vi "Teleop Drive subVI.vi"(9 "Buttons":bool[](array[boolean]), 10 "Axes":dbl[](array[numeric])) -> ()   [LabVIEW 2017]
doc: "This VI is called for each TeleOp packet received from the DS where the robot is not disabled. It is often used to read from the joysticks and update I/O or to update setpoints for timed control loops. It should complete and return within 20 milliseconds or it may miss DS packets."
uses:
  drive enum.ctl
  <vilib>/Rock Robotics/WPI/ThirdParty/Phoenix-LabVIEW/Motor Controller/Controls/CTRE_Phoenix_MotorControl_FeedbackDevice.ctl
  <vilib>/Rock Robotics/WPI/ThirdParty/Phoenix-LabVIEW/Motor Controller/Controls/CTRE_Phoenix_MotorControl_ControlMode.ctl
  <vilib>/Rock Robotics/WPI/Utilities/WPI_GetSetVariantRefNum.vi
  <vilib>/Rock Robotics/WPI/ThirdParty/Phoenix-LabVIEW/Motor Controller/Get/CTRE_Phoenix_MotorController_GetOutputCurrent_Enhanced.vi
  <vilib>/Rock Robotics/WPI/ThirdParty/Phoenix-LabVIEW/Motor Controller/Get/CTRE_Phoenix_MotorController_GetVoltage.vi
  <vilib>/Rock Robotics/WPI/ThirdParty/Phoenix-LabVIEW/Motor Controller/Get/CTRE_Phoenix_MotorController_GetClosedLoopData.vi
  <vilib>/Rock Robotics/WPI/ThirdParty/Phoenix-LabVIEW/Motor Controller/Get/CTRE_Phoenix_MotorController_GetSelectedSensorData.vi
  <vilib>/Rock Robotics/Network Tables/NT Write Variant.vi
  <vilib>/Rock Robotics/WPI/Solenoid/WPI_SolenoidSetEnum.vi
  <vilib>/Rock Robotics/WPI/Solenoid/WPI_SolenoidValue.ctl
panel:
  in  "X and Y values In":bool=TRUE
  in  "Tab Control":T1(tab)
  in  "Cruise Velocity 3":i32=2000
  in  "Max Acceleration 3":i32=2000
  in  "Cruise Velocity 4":i32=2000
  in  "Max Acceleration 4":i32=2000
  in  "P 3":dbl format="%#_13g"
  in  "I 3":dbl format="%#_13g"
  in  "D 3":dbl format="%#_13g"
  in  "F 3":dbl=0.0095 format="%#_13g"
  in  "P 4":dbl format="%#_13g"
  in  "I 4":dbl format="%#_13g"
  in  "D 4":dbl format="%#_13g"
  in  "F 4":dbl=0.0095 format="%#_13g"
  out "Velocity (Raw Sensor Units per 100 ms) 6":i32
  out "Position (inches) 6":i32
  out "Percent Output 4":dbl
  out "Velocity (Raw Sensor Units per 100 ms) 5":i32
  out "Position (Raw Sensor Units) 5":i32
  out "Percent Output 3":dbl
  out "Output Current 3":dbl
  out "Closed-loop Error 4":i32
  out "Output Current 4":dbl
  out "Closed-loop Error 3":i32
  out "Position (inches) 5":i32
  out "Position (Raw Sensor Units) 6":i32
  in  "P":dbl format="%#_13g"
  in  "I":dbl format="%#_13g"
  in  "D":dbl format="%#_13g"
  in  "F":dbl=0.0095 format="%#_13g"
  in  "Cruise Velocity":i32=2000
  in  "Max Acceleration":i32=2000
  in  "Cruise Velocity 2":i32=2000
  in  "Max Acceleration 2":i32=2000
  in  "P 2":dbl format="%#_13g"
  in  "I 2":dbl format="%#_13g"
  in  "D 2":dbl format="%#_13g"
  in  "F 2":dbl=0.0095 format="%#_13g"
  out "Closed-loop Error 2":i32
  out "Percent Output 2":dbl
  out "Output Current 2":dbl
  out "Velocity (Raw Sensor Units per 100 ms) 4":i32
  out "Position (Raw Sensor Units) 4":i32
  out "Percent Output":dbl
  out "Output Current":dbl
  out "Velocity (Raw Sensor Units per 100 ms) 3":i32
  out "Position (Raw Sensor Units) 3":i32
  out "Closed-loop Error":i32
  out "Velocity (Raw Sensor Units per 100 ms) 7":i32
  out "Position (Raw Sensor Units) 7":i32
  out "Closed-loop Error 5":i32
  out "Percent Output 5":dbl
  out "Output Current 5":dbl
  out "Closed-loop Error 6":i32
  in  "Cruise Velocity 5":i32=2000
  in  "Max Acceleration 5":i32=2000
  in  "Cruise Velocity 6":i32=2000
  in  "Max Acceleration 6":i32=2000
  in  "P 5":dbl format="%#_13g"
  in  "D 5":dbl format="%#_13g"
  in  "F 5":dbl=0.0095 format="%#_13g"
  in  "I 5":dbl format="%#_13g"
  in  "P 6":dbl format="%#_13g"
  in  "I 6":dbl format="%#_13g"
  in  "D 6":dbl format="%#_13g"
  in  "F 6":dbl=0.0095 format="%#_13g"
  out "Velocity (Raw Sensor Units per 100 ms) 8":i32
  out "Position (Raw Sensor Units) 8":i32
  out "Percent Output 6":dbl
  out "Output Current 6":dbl
  out "Position (Raw Sensor Units)":i32
  out "Velocity (Raw Sensor Units per 100 ms)":i32
  out "Position (Raw Sensor Units) 2":i32
  out "Velocity (Raw Sensor Units per 100 ms) 2":i32
  in  "X axis value":dbl
  in  "Y axis value":dbl
  out "encoder position":i32(graph)
  out "X and Y":T2(graph)
  out "joystick X":dbl
  out "joystick Y":dbl
  out "closed loop error":T3(graph)
  out "voltage vs current left":T2(graph)
  out "voltage vs current right":T2(graph)
  out "Speed Closed Loop Plots":T4(graph)
  # "front panel"
  # "joystick"
  # "what we want"
  # "actual"
  # "0.005740418607"
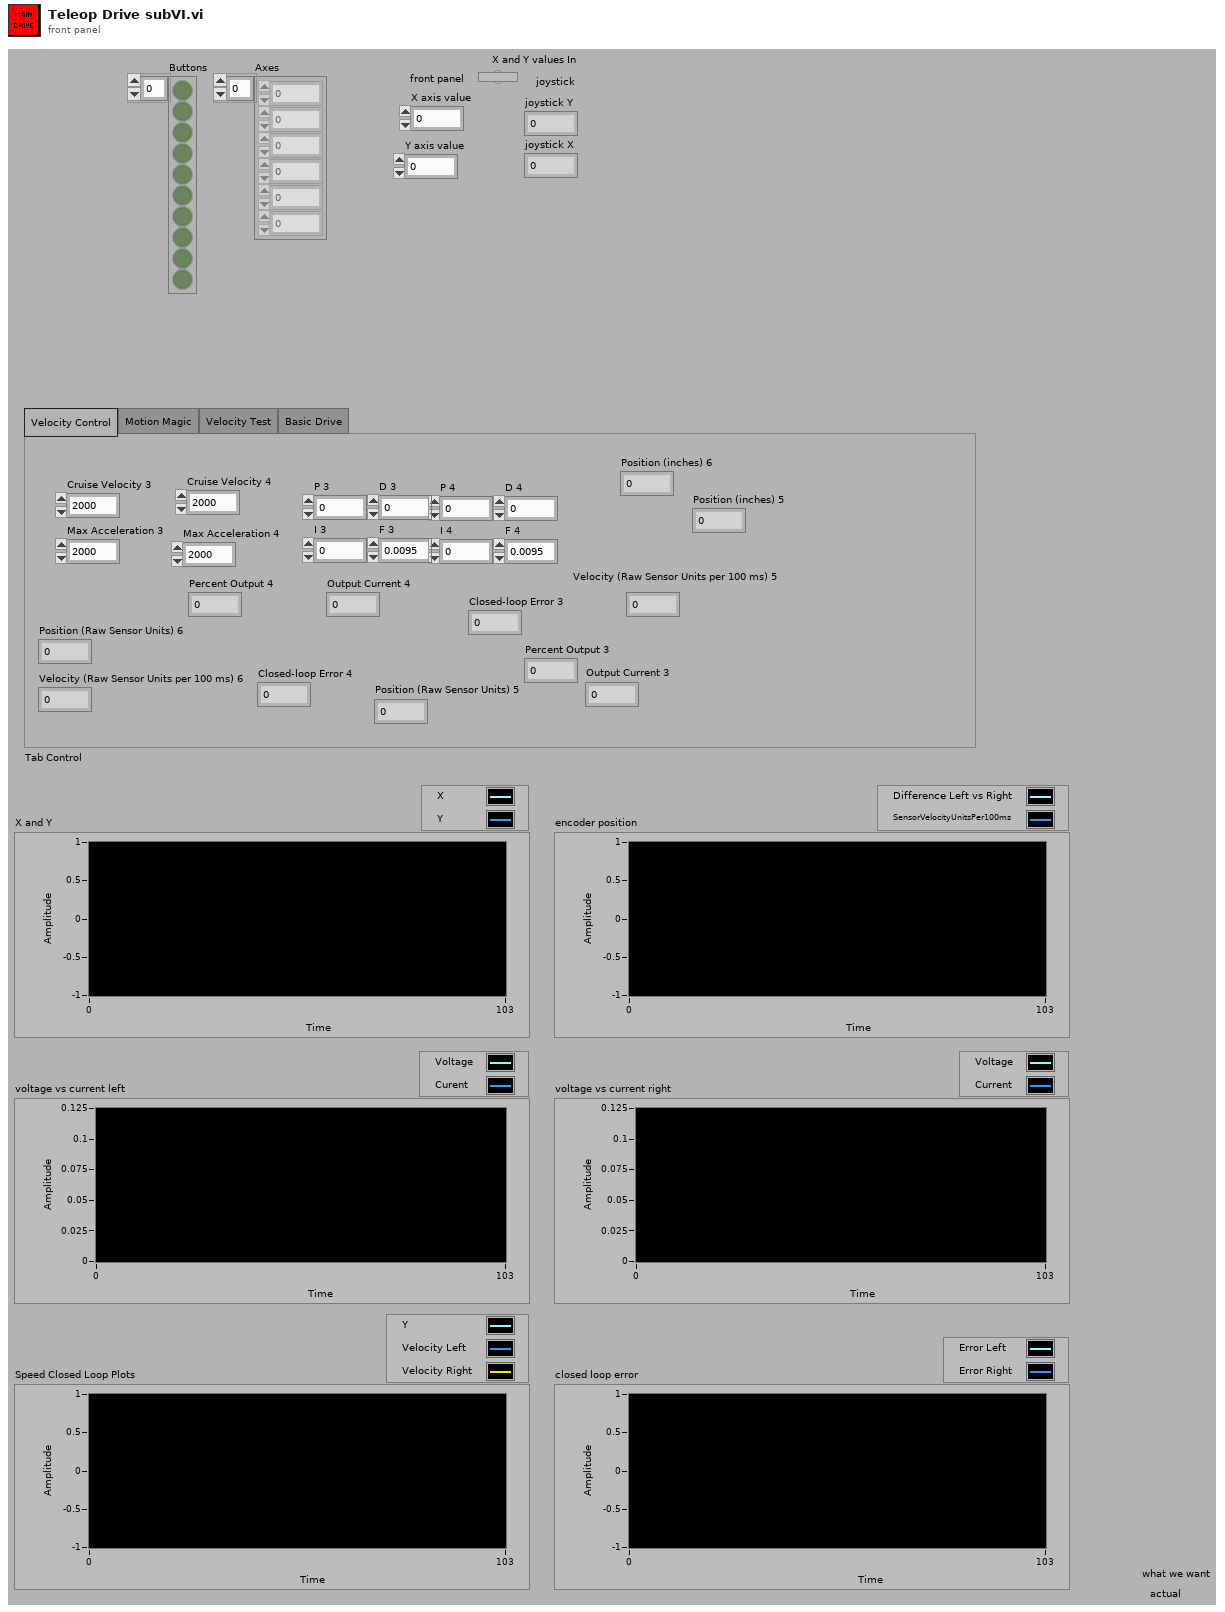
[diagram p1: front panel]
types:
  T1 = enum32{"Velocity Control", "Motion Magic", "Velocity Test", "Basic Drive"}
  T2 = cluster{"Percent Output":dbl, "Output Current":dbl}
  T3 = cluster{"Closed-loop Error":i32, "Closed-loop Error":i32}
  T4 = cluster{dbl, "Velocity (Raw Sensor Units per 100 ms)":i32, "Velocity (Raw Sensor Units per 100 ms)":i32}
  T5 = typedef "drive enum.ctl" = enum16{"Velocity Control", "Motion Magic", "Velocity Test", "Basic Drive"}
  T6 = typedef "WPI_SolenoidValue.ctl" = enum16{"Off", "On", "Forward", "Reverse"}
  T7 = typedef "WPI_SolenoidDevRef.ctl" = cluster{"DevStatus":errorcluster, "Pneumatics Control Module":u8, "Forward Solenoid Channel":T8, "Reverse Solenoid Channel":T8}
  T8 = typedef "WPI_SolenoidChannel.ctl" = enum8{"Solenoid 0", "Solenoid 1", "Solenoid 2", "Solenoid 3", "Solenoid 4", "Solenoid 5", "Solenoid 6", "Solenoid 7", "Invalid"}
  T9 = typedef "WPI_RobotDriveDevRef.ctl" = cluster{"DevStatus":errorcluster, "Motors[]":T10[], "Square Inputs":bool, "Max Output":dbl}
  T10 = typedef "WPI_MotorControlDeviceRef.ctl" = cluster{"DeviceStatus":errorcluster, "Type":T11, "PWM":cluster{"PWM Channel":T12, "DeadBand":T13}, "CAN":cluster{"Device Number":u8, "SetOutput VI Ref":variant, "GetOutput VI Ref":variant, "Enable VI Ref":variant, "Disable VI Ref":variant, "Data":variant}, "Invert":bool, "DIO PWM":cluster{"PWM \"Enable\" Channel":T12, "DIOChannel":T14, "PWM Rate":dbl}}
  T11 = typedef "WPI_MotorControlType.ctl" = enum16{"PWM", "CAN", "DIO PWM"}
  T12 = typedef "FPGA_DIOPWMChannel.ctl" = enum8{"PWM 0", "PWM 1", "PWM 2", "PWM 3", "PWM 4", "PWM 5", "PWM 6", "PWM 7", "PWM 8", "PWM 9", "PWM MXP 0", "PWM MXP 1", "PWM MXP 2", "PWM MXP 3", "PWM MXP 4", "PWM MXP 5", "PWM MXP 6", "PWM MXP 7", "PWM MXP 8", "PWM MXP 9", "Invalid"}
  T13 = typedef "WPI_PWMDeadband.ctl" = cluster{"Name":string, "maxPositivePwm":i32, "minPositivePwm":i32, "centerPwm":i32, "maxNegativePwm":i32, "minNegativePwm":i32, "angularRange":u16}
  T14 = typedef "FPGA_DIOChannel.ctl" = enum8{"DIO 0", "DIO 1", "DIO 2", "DIO 3", "DIO 4", "DIO 5", "DIO 6", "DIO 7", "DIO 8", "DIO 9", "DIO MXP 0", "DIO MXP 1", "DIO MXP 2", "DIO MXP 3", "DIO MXP 4", "DIO MXP 5", "DIO MXP 6", "DIO MXP 7", "DIO MXP 8", "DIO MXP 9", "DIO MXP 10", "DIO MXP 11", "DIO MXP 12", "DIO MXP 13", "DIO MXP 14", "DIO MXP 15", "SPI Port CS1", "SPI Port CS2", "SPI Port CS3", "SPI Port MISO", "SPI Port MOSI", "Invalid"}
  T15 = typedef "CTRE_Phoenix_MotorControl_ControlMode.ctl" = u16
  T16 = typedef "CTRE_Phoenix_MotorControl_FeedbackDevice.ctl" = i8
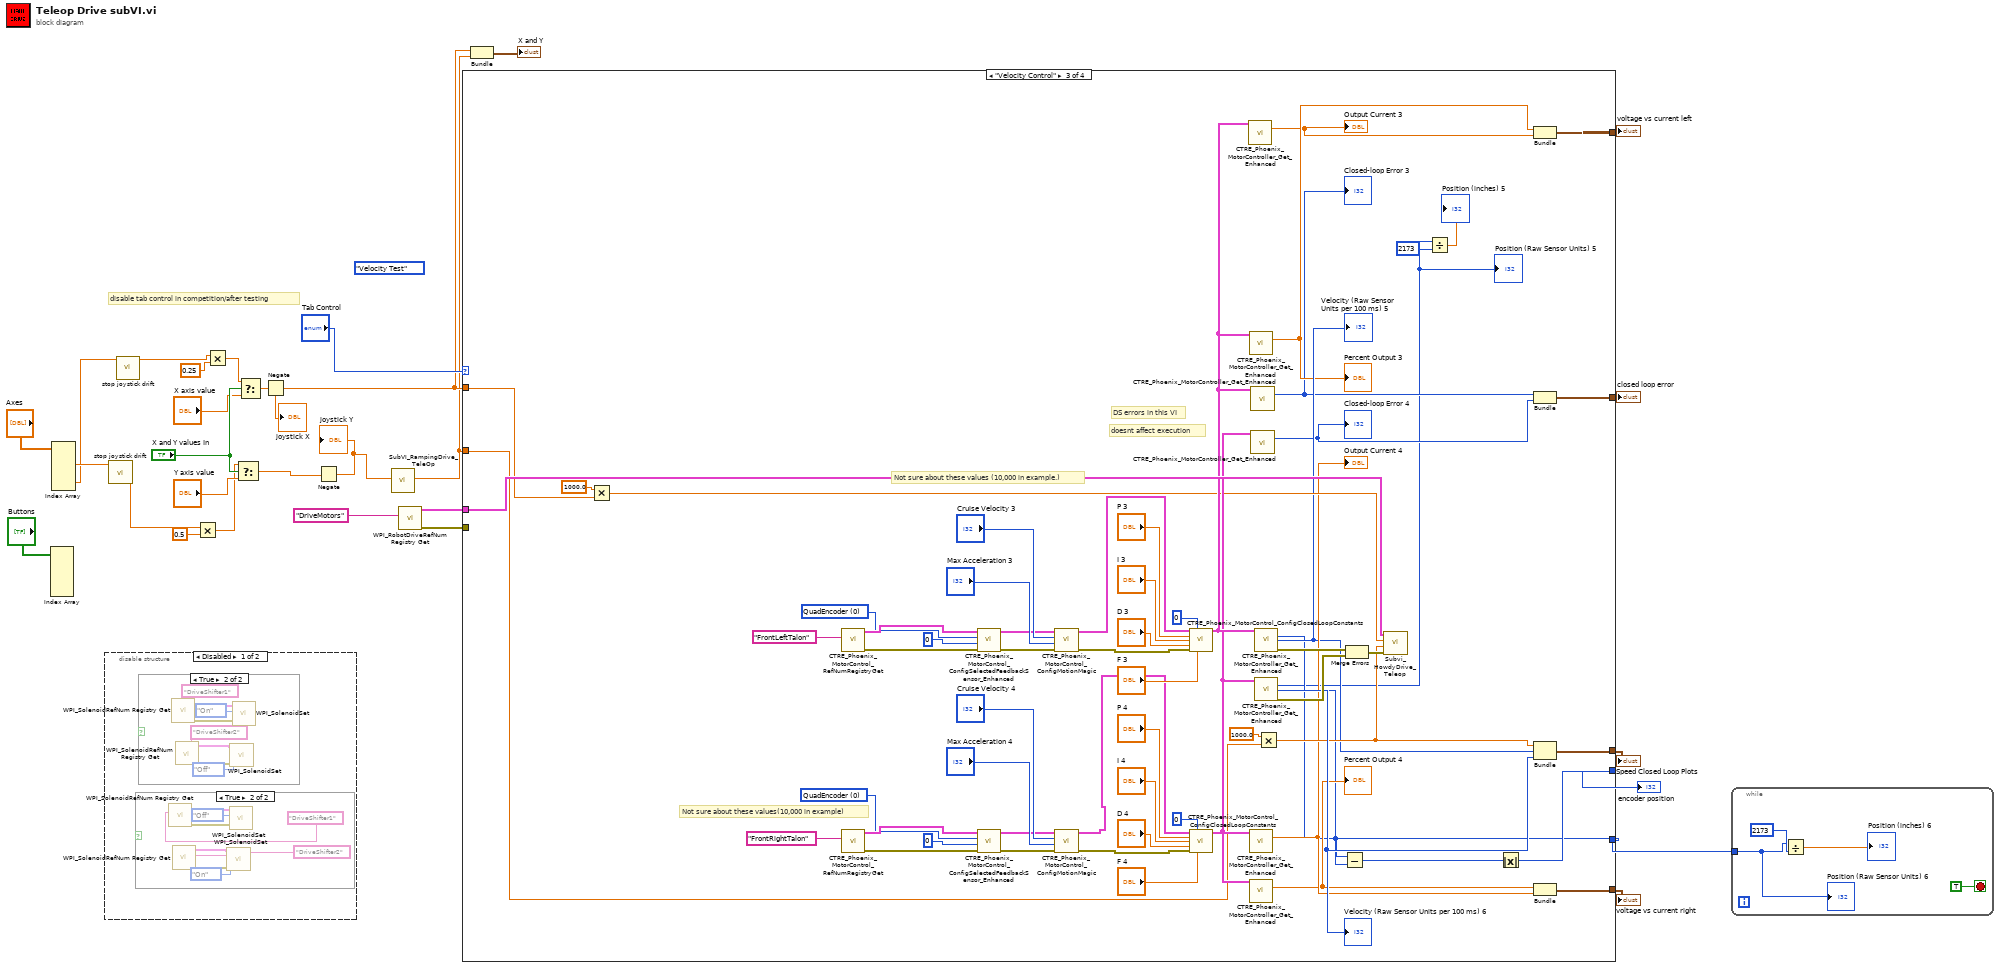
[diagram p0: block diagram]
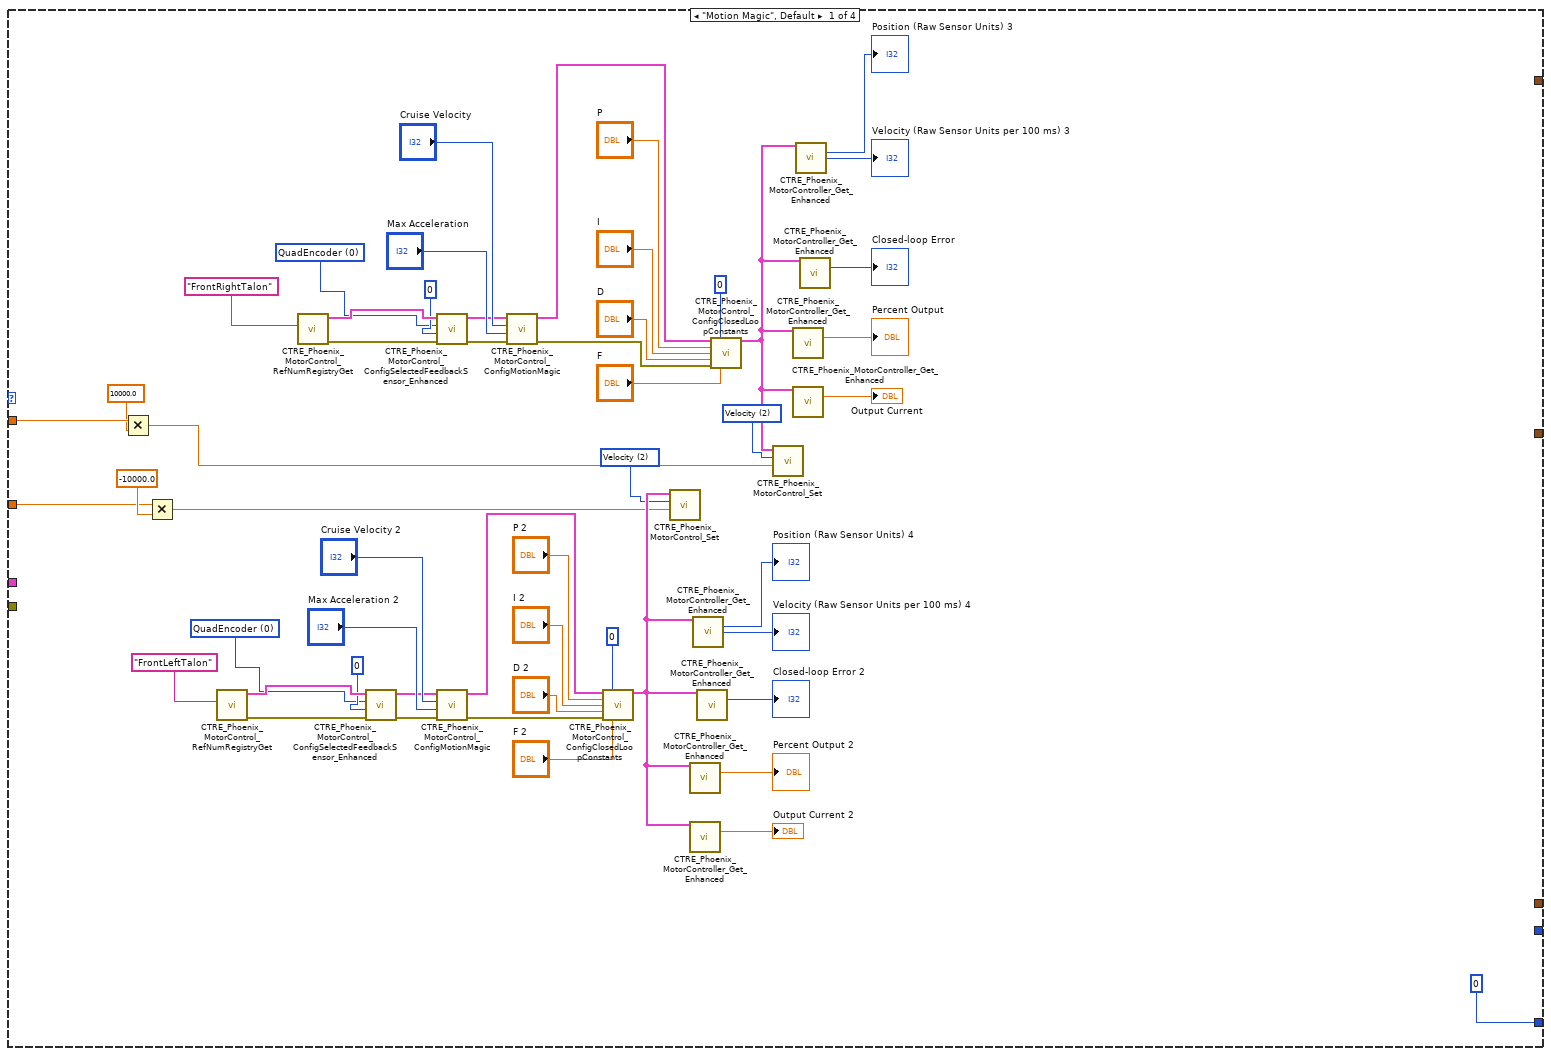
[diagram p5: hidden frame]
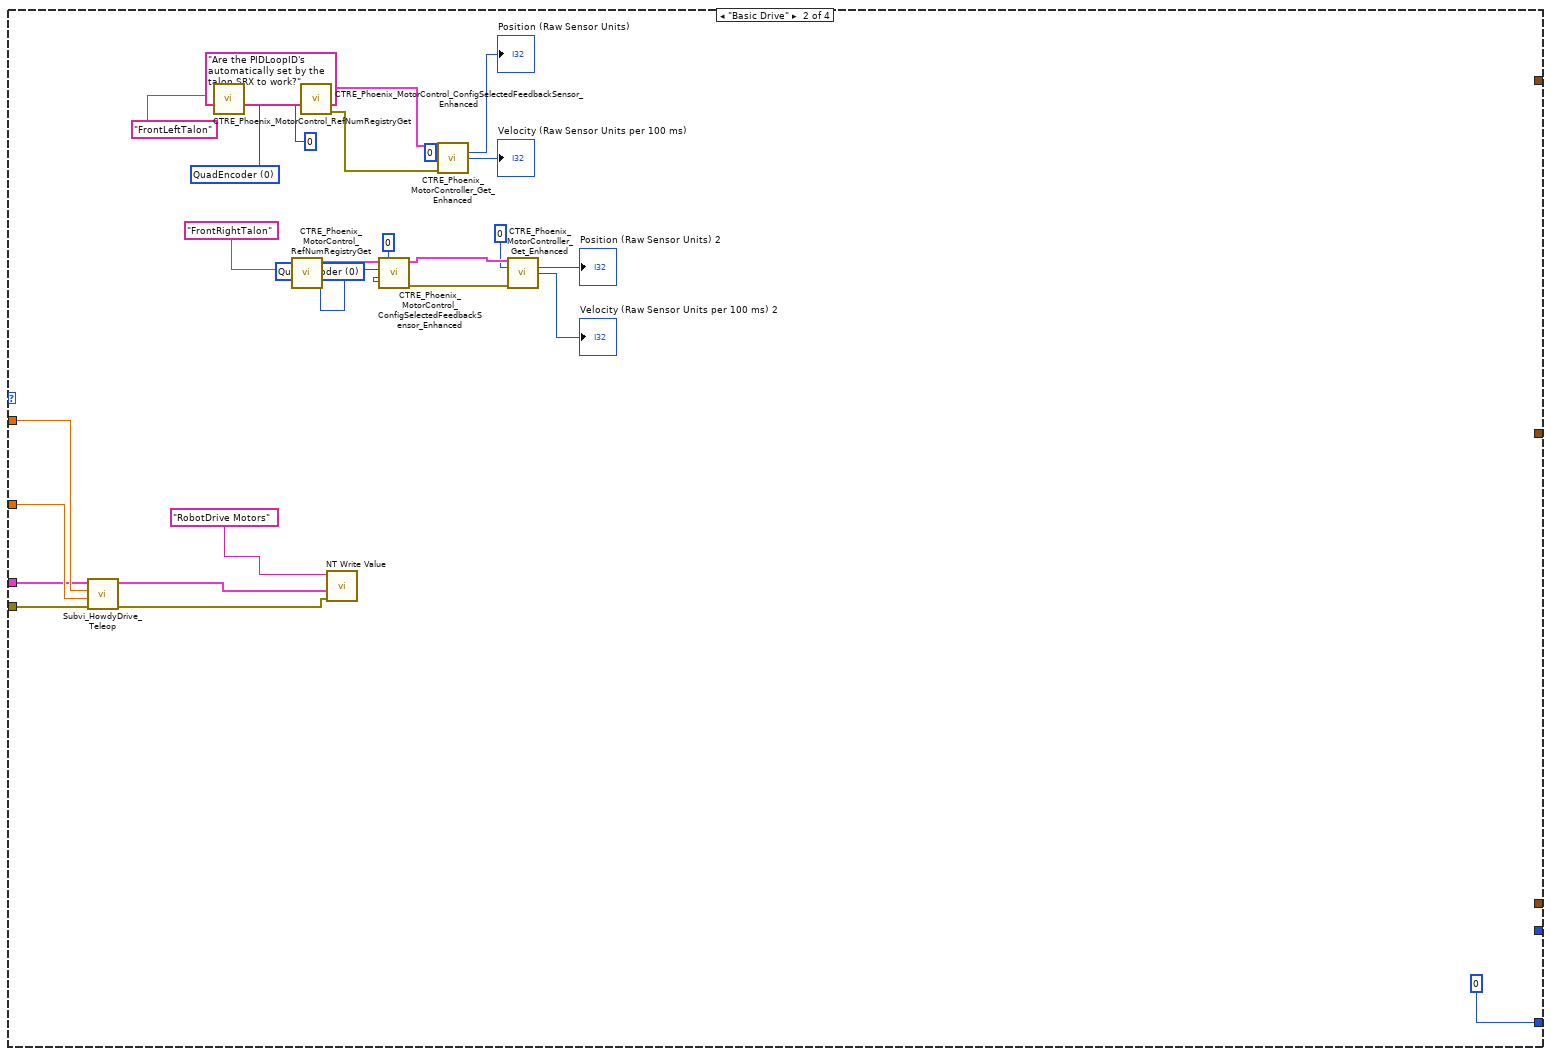
[diagram p6: hidden frame]
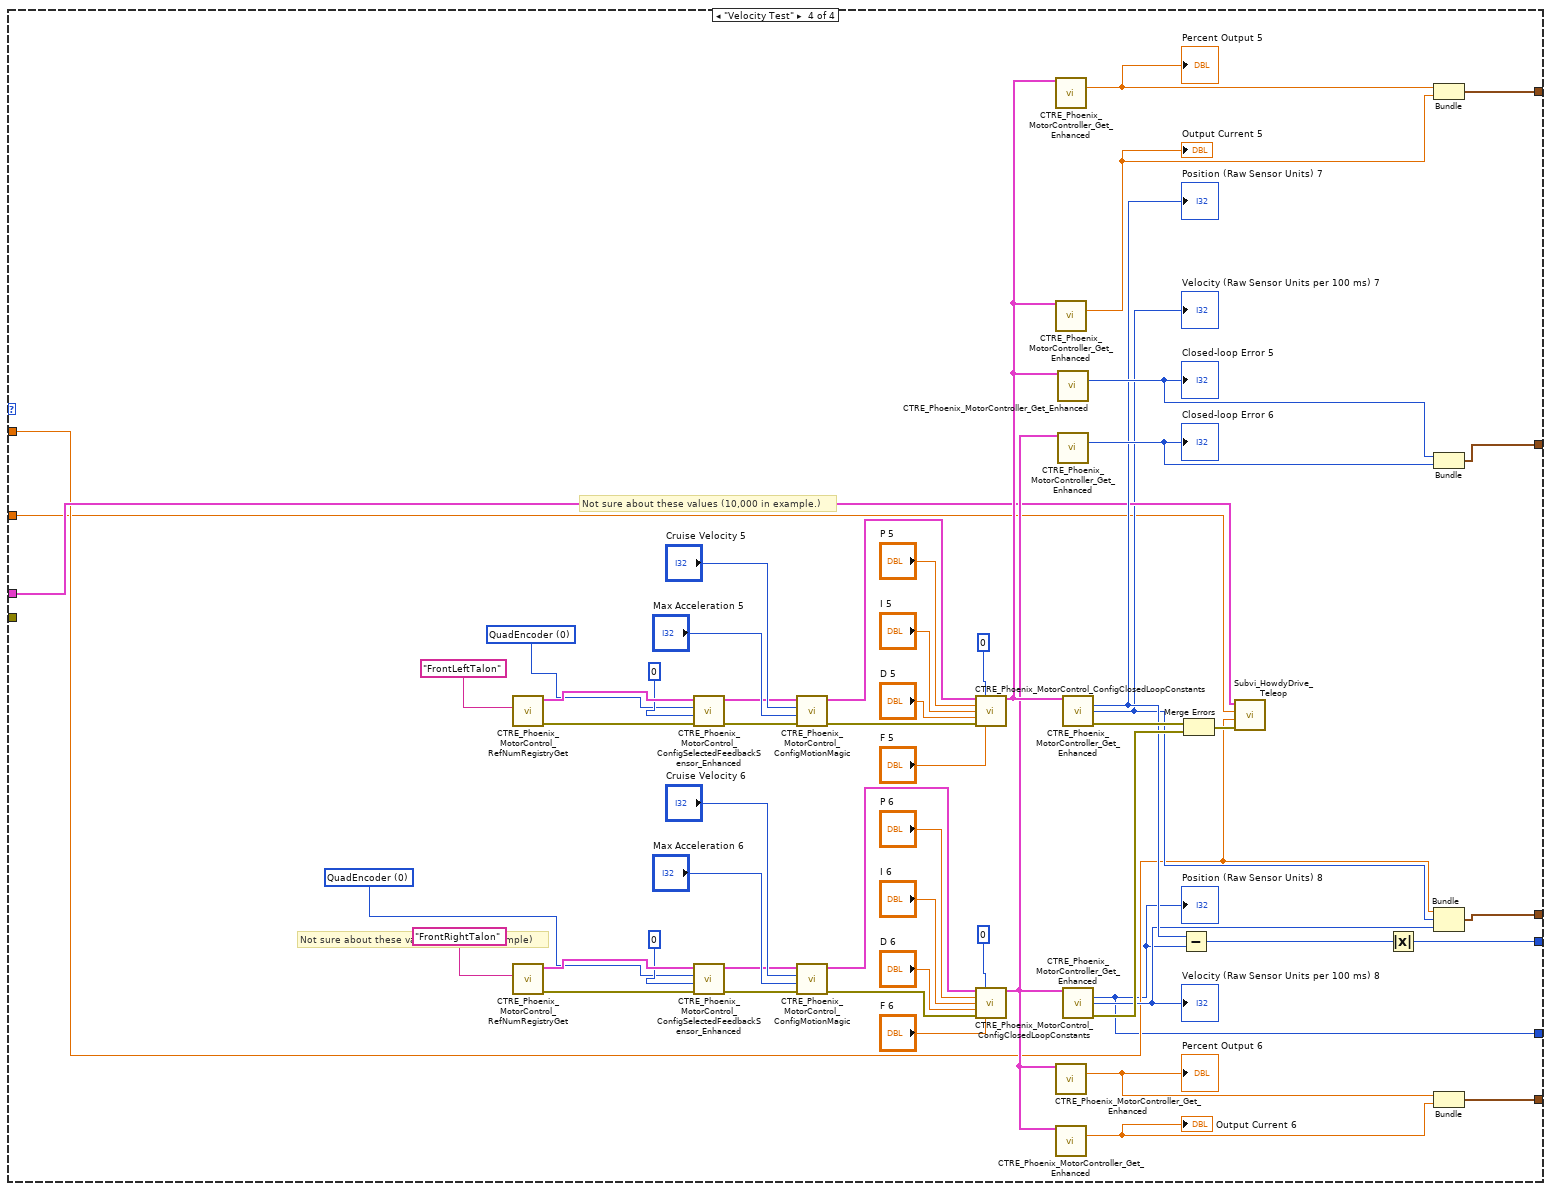
[diagram p7: hidden frame]
diagram:
  (unwired) drive_enum."Velocity Test"
  # "disable tab control in competition/after testing"
  n1 = Index Array(array="Buttons") -> ()  [unwired: 6 in, 6 out]
  n2 = Index Array(array="Axes") -> (element #2=w19:dbl, element #5=w12:dbl)  [unwired: 6 in, 4 out]
  n3 = disable-structure shown="Disabled" {
    frame Disabled {
      n4 = case shown="True" {
        selector: _ -> [_ _]
        frame False {
        }
        frame True {
          n5 = call <vilib>:"WPI_SolenoidRefNum Registry Get.vi"("refnum name"="DriveShifter1") -> ("error out"=w44:errorcluster, "SolenoidDevRef"=w45:T7)  [unwired: 9 in]
          n6 = call <vilib>:"WPI_SolenoidRefNum Registry Get.vi"("refnum name"="DriveShifter2") -> ("error out"=w42:errorcluster, "SolenoidDevRef"=w43:T7)  [unwired: 9 in]
          n7 = call-poly <vilib>:"WPI_SolenoidSet.vi"("error in (no error)"=w42, "Value"=WPI_SolenoidValue."On", "SolenoidDevRef"=w43) -> ()  [unwired: 7 in, 2 out]
          n8 = call-poly <vilib>:"WPI_SolenoidSet.vi"("error in (no error)"=w44, "Value"=WPI_SolenoidValue."Off", "SolenoidDevRef"=w45) -> ()  [unwired: 7 in, 2 out]
        }
      }
      n9 = case shown="True" {
        selector: _ -> [_ _]
        frame False {
        }
        frame True {
          n10 = call <vilib>:"WPI_SolenoidRefNum Registry Get.vi"("refnum name"="DriveShifter1") -> ("error out"=w36:errorcluster, "SolenoidDevRef"=w37:T7)  [unwired: 9 in]
          n11 = call <vilib>:"WPI_SolenoidRefNum Registry Get.vi"("refnum name"="DriveShifter2") -> ("error out"=w34:errorcluster, "SolenoidDevRef"=w35:T7)  [unwired: 9 in]
          n12 = call-poly <vilib>:"WPI_SolenoidSet.vi"("error in (no error)"=w34, "Value"=WPI_SolenoidValue."Off", "SolenoidDevRef"=w35) -> ()  [unwired: 7 in, 2 out]
          n13 = call-poly <vilib>:"WPI_SolenoidSet.vi"("error in (no error)"=w36, "Value"=WPI_SolenoidValue."On", "SolenoidDevRef"=w37) -> ()  [unwired: 7 in, 2 out]
        }
      }
    }
    frame Enabled {
    }
  }
  n14 = call "stop joystick drift.vi"("upper limit in"=w19) -> ("upper limit out"=w8:dbl)  [unwired: 10 in]
  n15 = call "stop joystick drift.vi"("upper limit in"=w12) -> ("upper limit out"=w10:dbl)  [unwired: 10 in]
  n16 = Multiply(x=w8, y=0.5) -> (x*y=w6:dbl)
  n17 = Multiply(x=w10, y=0.25) -> (x*y=w5:dbl)
  n18 = Select(t=w6, s="X and Y values In", f="Y axis value") -> (s? t:f=w16:dbl)
  n19 = Select(t=w5, s="X and Y values In", f="X axis value") -> (s? t:f=w17:dbl)
  n20 = Negate(x=w17) -> (-x=w13:dbl)
  "joystick X" <- w13
  n21 = Negate(x=w16) -> (-x=w1:dbl)
  "joystick Y" <- w1
  n22 = call "SubVI_RampingDrive_TeleOp.vi"("joystick Y Input"=w1) -> ("joystick Y Output"=w2:dbl)  [unwired: 9 in, 1 out]
  n23 = call <vilib>:"WPI_RobotDriveRefNum Registry Get.vi"("refnum name"="DriveMotors") -> ("error out"=w11:errorcluster, "RobotDriveDevRef"=w28:T9)  [unwired: 1 in, 8 out]
  n24 = case shown="\"Velocity Control\"" "Tab Control" {
    tunnel: w2 -> [w49 w123 w149 w188]
    tunnel: w13 -> [w52 w122 w150 w189]
    tunnel: w28 -> [_ w121 w186 w197]
    tunnel: [_ _ w137 w196] -> w26
    tunnel: [_ _ w135 w194] -> w25
    tunnel: [_ _ w134 w192] -> w24
    tunnel: [_ _ w133 w193] -> w23
    tunnel: [_ _ w136 w195] -> w22
    tunnel: w11 -> [_ w101 _ _]
    tunnel: [0 ("Position (Raw Sensor Units)") 0 ("Position (Raw Sensor Units)") w128 w187] -> w4
    frame "Motion Magic", Default {
      w57 = T15 2 items=["PercentOutput"=0, "Position"=1, "Velocity"=2, "Current"=3, "Follower"=5, "MotionProfile"=6, "MotionMagic"=7, "MotionMagicArc"=8, "MotionProfileArc"=10, "Disabled"=15] ("Control Mode")
      w54 = T16 0 items=["None"=-1, "QuadEncoder"=0, "Analog"=2, "Tachometer"=4, "Pulse Width Encoded Position"=8, "Sensor Sum (S0 + S1)"=9, "Sensor Difference (D0 - D1)"=10, "Remote Source 0"=11, "Remote Source 1"=12, "Software Emulated"=15] ("Feedback Device")
      w80 = T15 2 items=["PercentOutput"=0, "Position"=1, "Velocity"=2, "Current"=3, "Follower"=5, "MotionProfile"=6, "MotionMagic"=7, "MotionMagicArc"=8, "MotionProfileArc"=10, "Disabled"=15] ("Control Mode")
      w77 = T16 0 items=["None"=-1, "QuadEncoder"=0, "Analog"=2, "Tachometer"=4, "Pulse Width Encoded Position"=8, "Sensor Sum (S0 + S1)"=9, "Sensor Difference (D0 - D1)"=10, "Remote Source 0"=11, "Remote Source 1"=12, "Software Emulated"=15] ("Feedback Device")
      n25 = Multiply(x=w52, y=10000.0) -> (x*y=w47:dbl)
      n26 = Multiply(x=w49, y=-10000.0) -> (x*y=w48:dbl)
      n27 = call <vilib>:"CTRE_Phoenix_MotorControl_RefNumRegistryGet.vi"("refnum name"="FrontLeftTalon") -> ("error out"=w82:errorcluster, "PhoenixMotorControlDevRef"=w81:T10)  [unwired: 9 in]
      n28 = call <vilib>:"CTRE_Phoenix_MotorControl_RefNumRegistryGet.vi"("refnum name"="FrontRightTalon") -> ("error out"=w59:errorcluster, "PhoenixMotorControlDevRef"=w58:T10)  [unwired: 9 in]
      n29 = call <vilib>:"CTRE_Phoenix_MotorControl_ConfigSelectedFeedbackSensor_Enhanced.vi"("error in (no error)"=w82, "pidLoopIdx"=0, "Feedback Device"=w77, "PhoenixMotorControlDevRef"=w81) -> ("error out"=w84:errorcluster, "PhoenixMotorControlDevRef"=w83:T10)  [unwired: 6 in]
      n30 = call <vilib>:"CTRE_Phoenix_MotorControl_ConfigSelectedFeedbackSensor_Enhanced.vi"("error in (no error)"=w59, "pidLoopIdx"=0, "Feedback Device"=w54, "PhoenixMotorControlDevRef"=w58) -> ("error out"=w61:errorcluster, "PhoenixMotorControlDevRef"=w60:T10)  [unwired: 6 in]
      n31 = call <vilib>:"CTRE_Phoenix_MotorControl_ConfigMotionMagic.vi"("error in (no error)"=w84, "Acceleration"="Max Acceleration 2", "Cruise Velocity"="Cruise Velocity 2", "PhoenixMotorControlDevRef"=w83) -> ("error out"=w95:errorcluster, "PhoenixMotorControlDevRef"=w94:T10)  [unwired: 6 in]
      n32 = call <vilib>:"CTRE_Phoenix_MotorControl_ConfigMotionMagic.vi"("error in (no error)"=w61, "Acceleration"="Max Acceleration", "Cruise Velocity"="Cruise Velocity", "PhoenixMotorControlDevRef"=w60) -> ("error out"=w63:errorcluster, "PhoenixMotorControlDevRef"=w62:T10)  [unwired: 6 in]
      n33 = call <vilib>:"CTRE_Phoenix_MotorControl_ConfigClosedLoopConstants.vi"("PhoenixMotorControlDevRef"=w94, "slotIdx"=0, "P"="P 2", "I"="I 2", "D"="D 2", "error in (no error)"=w95, "F"="F 2") -> ("PhoenixMotorControlDevRef"=w98:T10)  [unwired: 7 in, 1 out]
      n34 = call <vilib>:"CTRE_Phoenix_MotorControl_Set.vi"("Output"=w48, "Control Mode"=w80, "PhoenixMotorControlDevRef"=w98) -> ()  [unwired: 7 in, 2 out]
      n35 = call-poly <vilib>:"CTRE_Phoenix_MotorController_Get_Enhanced.vi"("PhoenixMotorControlDevRef"=w98) -> ("Percent Output"=→"Percent Output 2":dbl)  [unwired: 10 in, 4 out]
      n36 = call-poly <vilib>:"CTRE_Phoenix_MotorController_Get_Enhanced.vi"("PhoenixMotorControlDevRef"=w98) -> ("Output Current"=→"Output Current 2":dbl)  [unwired: 12 in, 2 out]
      n37 = call-poly <vilib>:"CTRE_Phoenix_MotorController_Get_Enhanced.vi"("PhoenixMotorControlDevRef"=w98) -> ("Position (Raw Sensor Units)"=→"Position (Raw Sensor Units) 4":i32, "Velocity (Raw Sensor Units per 100 ms)"=→"Velocity (Raw Sensor Units per 100 ms) 4":i32)  [unwired: 11 in, 2 out]
      n38 = call-poly <vilib>:"CTRE_Phoenix_MotorController_Get_Enhanced.vi"("PhoenixMotorControlDevRef"=w98) -> ("Closed-loop Error"=→"Closed-loop Error 2":i32)  [unwired: 9 in, 5 out]
      n39 = call <vilib>:"CTRE_Phoenix_MotorControl_ConfigClosedLoopConstants.vi"("PhoenixMotorControlDevRef"=w62, "slotIdx"=0, "P"="P", "I"="I", "D"="D", "error in (no error)"=w63, "F"="F") -> ("PhoenixMotorControlDevRef"=w75:T10)  [unwired: 7 in, 1 out]
      n40 = call <vilib>:"CTRE_Phoenix_MotorControl_Set.vi"("Output"=w47, "Control Mode"=w57, "PhoenixMotorControlDevRef"=w75) -> ()  [unwired: 7 in, 2 out]
      n41 = call-poly <vilib>:"CTRE_Phoenix_MotorController_Get_Enhanced.vi"("PhoenixMotorControlDevRef"=w75) -> ("Percent Output"=→"Percent Output":dbl)  [unwired: 10 in, 4 out]
      n42 = call-poly <vilib>:"CTRE_Phoenix_MotorController_Get_Enhanced.vi"("PhoenixMotorControlDevRef"=w75) -> ("Output Current"=→"Output Current":dbl)  [unwired: 12 in, 2 out]
      n43 = call-poly <vilib>:"CTRE_Phoenix_MotorController_Get_Enhanced.vi"("PhoenixMotorControlDevRef"=w75) -> ("Position (Raw Sensor Units)"=→"Position (Raw Sensor Units) 3":i32, "Velocity (Raw Sensor Units per 100 ms)"=→"Velocity (Raw Sensor Units per 100 ms) 3":i32)  [unwired: 11 in, 2 out]
      n44 = call-poly <vilib>:"CTRE_Phoenix_MotorController_Get_Enhanced.vi"("PhoenixMotorControlDevRef"=w75) -> ("Closed-loop Error"=→"Closed-loop Error":i32)  [unwired: 9 in, 5 out]
    }
    frame "Basic Drive" {
      (unwired) "Are the PIDLoopID's automatically set by the talon SRX to work?"
      w112 = T16 0 items=["None"=-1, "QuadEncoder"=0, "Analog"=2, "Tachometer"=4, "Pulse Width Encoded Position"=8, "Sensor Sum (S0 + S1)"=9, "Sensor Difference (D0 - D1)"=10, "Remote Source 0"=11, "Remote Source 1"=12, "Software Emulated"=15] ("Feedback Device")
      w119 = T16 0 items=["None"=-1, "QuadEncoder"=0, "Analog"=2, "Tachometer"=4, "Pulse Width Encoded Position"=8, "Sensor Sum (S0 + S1)"=9, "Sensor Difference (D0 - D1)"=10, "Remote Source 0"=11, "Remote Source 1"=12, "Software Emulated"=15] ("Feedback Device")
      n45 = call "Subvi_HowdyDrive_Teleop.vi"("error in (no error)"=w101, "Y axis value"=w123, "X axis value"=w122, "RobotDriveDevRef"=w121) -> ("error out"=w100:errorcluster, "RobotDriveDevRef 2"=w124:T9)  [unwired: 6 in]
      n46 = call <vilib>:"CTRE_Phoenix_MotorControl_RefNumRegistryGet.vi"("refnum name"="FrontLeftTalon") -> ("PhoenixMotorControlDevRef"=w113:T10)  [unwired: 9 in, 1 out]
      n47 = call <vilib>:"CTRE_Phoenix_MotorControl_RefNumRegistryGet.vi"("refnum name"="FrontRightTalon") -> ("PhoenixMotorControlDevRef"=w105:T10)  [unwired: 9 in, 1 out]
      n48 = call <vilib>:"CTRE_Phoenix_MotorControl_ConfigSelectedFeedbackSensor_Enhanced.vi"("pidLoopIdx"=0, "Feedback Device"=w119, "PhoenixMotorControlDevRef"=w113) -> ("error out"=w117:errorcluster, "PhoenixMotorControlDevRef"=w118:T10)  [unwired: 7 in]
      n49 = call-poly <vilib>:"NT Write Value.vi"("error in"=w100, "Variant"=w124, "Name"="RobotDrive Motors") -> ()  [unwired: 8 in, 1 out]
      n50 = call <vilib>:"CTRE_Phoenix_MotorControl_ConfigSelectedFeedbackSensor_Enhanced.vi"("pidLoopIdx"=0, "Feedback Device"=w112, "PhoenixMotorControlDevRef"=w105) -> ("error out"=w110:errorcluster, "PhoenixMotorControlDevRef"=w111:T10)  [unwired: 7 in]
      n51 = call-poly <vilib>:"CTRE_Phoenix_MotorController_Get_Enhanced.vi"("PhoenixMotorControlDevRef"=w118, "pidLoopIdx"=u32 0, "error in"=w117) -> ("Position (Raw Sensor Units)"=→"Position (Raw Sensor Units)":i32, "Velocity (Raw Sensor Units per 100 ms)"=→"Velocity (Raw Sensor Units per 100 ms)":i32)  [unwired: 9 in, 2 out]
      n52 = call-poly <vilib>:"CTRE_Phoenix_MotorController_Get_Enhanced.vi"("PhoenixMotorControlDevRef"=w111, "pidLoopIdx"=u32 0, "error in"=w110) -> ("Position (Raw Sensor Units)"=→"Position (Raw Sensor Units) 2":i32, "Velocity (Raw Sensor Units per 100 ms)"=→"Velocity (Raw Sensor Units per 100 ms) 2":i32)  [unwired: 9 in, 2 out]
    }
    frame "Velocity Control" {
      w157 = T16 0 items=["None"=-1, "QuadEncoder"=0, "Analog"=2, "Tachometer"=4, "Pulse Width Encoded Position"=8, "Sensor Sum (S0 + S1)"=9, "Sensor Difference (D0 - D1)"=10, "Remote Source 0"=11, "Remote Source 1"=12, "Software Emulated"=15] ("Feedback Device")
      w172 = T16 0 items=["None"=-1, "QuadEncoder"=0, "Analog"=2, "Tachometer"=4, "Pulse Width Encoded Position"=8, "Sensor Sum (S0 + S1)"=9, "Sensor Difference (D0 - D1)"=10, "Remote Source 0"=11, "Remote Source 1"=12, "Software Emulated"=15] ("Feedback Device")
      # "doesnt affect execution"
      # "DS errors in this VI"
      # "Not sure about these values (10,000 in example.)"
      # "Not sure about these values(10,000 in example)"
      n53 = Multiply(x=1000.0, y=w150) -> (x*y=w148:dbl)
      n54 = call <vilib>:"CTRE_Phoenix_MotorControl_RefNumRegistryGet.vi"("refnum name"="FrontLeftTalon") -> ("error out"=w176:errorcluster, "PhoenixMotorControlDevRef"=w175:T10)  [unwired: 9 in]
      n55 = call <vilib>:"CTRE_Phoenix_MotorControl_RefNumRegistryGet.vi"("refnum name"="FrontRightTalon") -> ("error out"=w161:errorcluster, "PhoenixMotorControlDevRef"=w160:T10)  [unwired: 9 in]
      n56 = call <vilib>:"CTRE_Phoenix_MotorControl_ConfigSelectedFeedbackSensor_Enhanced.vi"("error in (no error)"=w176, "pidLoopIdx"=0, "Feedback Device"=w172, "PhoenixMotorControlDevRef"=w175) -> ("error out"=w178:errorcluster, "PhoenixMotorControlDevRef"=w177:T10)  [unwired: 6 in]
      n57 = call <vilib>:"CTRE_Phoenix_MotorControl_ConfigSelectedFeedbackSensor_Enhanced.vi"("error in (no error)"=w161, "pidLoopIdx"=0, "Feedback Device"=w157, "PhoenixMotorControlDevRef"=w160) -> ("error out"=w163:errorcluster, "PhoenixMotorControlDevRef"=w162:T10)  [unwired: 6 in]
      n58 = call <vilib>:"CTRE_Phoenix_MotorControl_ConfigMotionMagic.vi"("error in (no error)"=w178, "Acceleration"="Max Acceleration 3", "Cruise Velocity"="Cruise Velocity 3", "PhoenixMotorControlDevRef"=w177) -> ("error out"=w131:errorcluster, "PhoenixMotorControlDevRef"=w132:T10)  [unwired: 6 in]
      n59 = call <vilib>:"CTRE_Phoenix_MotorControl_ConfigMotionMagic.vi"("error in (no error)"=w163, "Acceleration"="Max Acceleration 4", "Cruise Velocity"="Cruise Velocity 4", "PhoenixMotorControlDevRef"=w162) -> ("error out"=w130:errorcluster, "PhoenixMotorControlDevRef"=w129:T10)  [unwired: 6 in]
      n60 = call <vilib>:"CTRE_Phoenix_MotorControl_ConfigClosedLoopConstants.vi"("PhoenixMotorControlDevRef"=w132, "slotIdx"=0, "P"="P 3", "I"="I 3", "D"="D 3", "error in (no error)"=w131, "F"="F 3") -> ("PhoenixMotorControlDevRef"=w185:T10)  [unwired: 7 in, 1 out]
      n61 = call <vilib>:"CTRE_Phoenix_MotorControl_ConfigClosedLoopConstants.vi"("PhoenixMotorControlDevRef"=w129, "slotIdx"=0, "P"="P 4", "I"="I 4", "D"="D 4", "error in (no error)"=w130, "F"="F 4") -> ("PhoenixMotorControlDevRef"=w170:T10)  [unwired: 7 in, 1 out]
      n62 = call-poly <vilib>:"CTRE_Phoenix_MotorController_Get_Enhanced.vi"("PhoenixMotorControlDevRef"=w185) -> ("Output Current"=w141:dbl)  [unwired: 12 in, 2 out]
      "Output Current 3" <- w141
      n63 = call-poly <vilib>:"CTRE_Phoenix_MotorController_Get_Enhanced.vi"("PhoenixMotorControlDevRef"=w185) -> ("Percent Output"=w142:dbl)  [unwired: 10 in, 4 out]
      "Percent Output 3" <- w142
      n64 = call-poly <vilib>:"CTRE_Phoenix_MotorController_Get_Enhanced.vi"("PhoenixMotorControlDevRef"=w170) -> ("Output Current"=w145:dbl)  [unwired: 12 in, 2 out]
      "Output Current 4" <- w145
      n65 = call-poly <vilib>:"CTRE_Phoenix_MotorController_Get_Enhanced.vi"("PhoenixMotorControlDevRef"=w170) -> ("Percent Output"=w144:dbl)  [unwired: 10 in, 4 out]
      "Percent Output 4" <- w144
      n66 = call-poly <vilib>:"CTRE_Phoenix_MotorController_Get_Enhanced.vi"("PhoenixMotorControlDevRef"=w185) -> ("Closed-loop Error"=w140:i32)  [unwired: 9 in, 5 out]
      "Closed-loop Error 3" <- w140
      n67 = call-poly <vilib>:"CTRE_Phoenix_MotorController_Get_Enhanced.vi"("PhoenixMotorControlDevRef"=w170) -> ("Closed-loop Error"=w139:i32)  [unwired: 9 in, 5 out]
      "Closed-loop Error 4" <- w139
      n68 = call-poly <vilib>:"CTRE_Phoenix_MotorController_Get_Enhanced.vi"("PhoenixMotorControlDevRef"=w185) -> ("Position (Raw Sensor Units)"=w128:i32, "Velocity (Raw Sensor Units per 100 ms)"=w143:i32, "error out"=w154:errorcluster)  [unwired: 11 in, 1 out]
      "Velocity (Raw Sensor Units per 100 ms) 5" <- w143
      n69 = call-poly <vilib>:"CTRE_Phoenix_MotorController_Get_Enhanced.vi"("PhoenixMotorControlDevRef"=w170) -> ("Position (Raw Sensor Units)"=w125:i32, "Velocity (Raw Sensor Units per 100 ms)"=w147:i32, "error out"=w155:errorcluster)  [unwired: 11 in, 1 out]
      "Position (Raw Sensor Units) 5" <- w125
      "Velocity (Raw Sensor Units per 100 ms) 6" <- w147
      n70 = Multiply(x=1000.0, y=w149) -> (x*y=w146:dbl)
      n71 = Subtract(x=w128, y=w125) -> (x-y=w138:i32)
      n72 = Merge Errors(w154, w155) -> (w153:errorcluster)
      n73 = call "Subvi_HowdyDrive_Teleop.vi"("error in (no error)"=w153, "Y axis value"=w146, "X axis value"=w148, "RobotDriveDevRef"=w186) -> ()  [unwired: 6 in, 2 out]
      n74 = Divide(x=w125, y=2173) -> (x/y=→"Position (inches) 5":dbl)
      n75 = Absolute Value(x=w138) -> (abs(x)=w137:i32)
      n76 = Bundle("Percent Output"=w142, "Output Current"=w141) -> (w135:T2)  [unwired: 1 in]
      n77 = Bundle("Closed-loop Error"=w140, "Closed-loop Error"=w139) -> (w136:T3)  [unwired: 1 in]
      n78 = Bundle(w146, "Velocity (Raw Sensor Units per 100 ms)"=w143, "Velocity (Raw Sensor Units per 100 ms)"=w147) -> (w134:T4)  [unwired: 1 in]
      n79 = Bundle("Percent Output"=w144, "Output Current"=w145) -> (w133:T2)  [unwired: 1 in]
    }
    frame "Velocity Test" {
      w210 = T16 0 items=["None"=-1, "QuadEncoder"=0, "Analog"=2, "Tachometer"=4, "Pulse Width Encoded Position"=8, "Sensor Sum (S0 + S1)"=9, "Sensor Difference (D0 - D1)"=10, "Remote Source 0"=11, "Remote Source 1"=12, "Software Emulated"=15] ("Feedback Device")
      w227 = T16 0 items=["None"=-1, "QuadEncoder"=0, "Analog"=2, "Tachometer"=4, "Pulse Width Encoded Position"=8, "Sensor Sum (S0 + S1)"=9, "Sensor Difference (D0 - D1)"=10, "Remote Source 0"=11, "Remote Source 1"=12, "Software Emulated"=15] ("Feedback Device")
      # "Not sure about these values (10,000 in example.)"
      # "Not sure about these values(10,000 in example)"
      n80 = call <vilib>:"CTRE_Phoenix_MotorControl_RefNumRegistryGet.vi"("refnum name"="FrontLeftTalon") -> ("error out"=w231:errorcluster, "PhoenixMotorControlDevRef"=w230:T10)  [unwired: 9 in]
      n81 = call <vilib>:"CTRE_Phoenix_MotorControl_RefNumRegistryGet.vi"("refnum name"="FrontRightTalon") -> ("error out"=w214:errorcluster, "PhoenixMotorControlDevRef"=w213:T10)  [unwired: 9 in]
      n82 = call <vilib>:"CTRE_Phoenix_MotorControl_ConfigSelectedFeedbackSensor_Enhanced.vi"("error in (no error)"=w231, "pidLoopIdx"=0, "Feedback Device"=w227, "PhoenixMotorControlDevRef"=w230) -> ("error out"=w233:errorcluster, "PhoenixMotorControlDevRef"=w232:T10)  [unwired: 6 in]
      n83 = call <vilib>:"CTRE_Phoenix_MotorControl_ConfigSelectedFeedbackSensor_Enhanced.vi"("error in (no error)"=w214, "pidLoopIdx"=0, "Feedback Device"=w210, "PhoenixMotorControlDevRef"=w213) -> ("error out"=w216:errorcluster, "PhoenixMotorControlDevRef"=w215:T10)  [unwired: 6 in]
      n84 = call <vilib>:"CTRE_Phoenix_MotorControl_ConfigMotionMagic.vi"("error in (no error)"=w233, "Acceleration"="Max Acceleration 5", "Cruise Velocity"="Cruise Velocity 5", "PhoenixMotorControlDevRef"=w232) -> ("error out"=w239:errorcluster, "PhoenixMotorControlDevRef"=w238:T10)  [unwired: 6 in]
      n85 = call <vilib>:"CTRE_Phoenix_MotorControl_ConfigMotionMagic.vi"("error in (no error)"=w216, "Acceleration"="Max Acceleration 6", "Cruise Velocity"="Cruise Velocity 6", "PhoenixMotorControlDevRef"=w215) -> ("error out"=w218:errorcluster, "PhoenixMotorControlDevRef"=w217:T10)  [unwired: 6 in]
      n86 = call <vilib>:"CTRE_Phoenix_MotorControl_ConfigClosedLoopConstants.vi"("PhoenixMotorControlDevRef"=w238, "slotIdx"=0, "P"="P 5", "I"="I 5", "D"="D 5", "error in (no error)"=w239, "F"="F 5") -> ("PhoenixMotorControlDevRef"=w242:T10)  [unwired: 7 in, 1 out]
      n87 = call <vilib>:"CTRE_Phoenix_MotorControl_ConfigClosedLoopConstants.vi"("PhoenixMotorControlDevRef"=w217, "slotIdx"=0, "P"="P 6", "I"="I 6", "D"="D 6", "error in (no error)"=w218, "F"="F 6") -> ("PhoenixMotorControlDevRef"=w225:T10)  [unwired: 7 in, 1 out]
      n88 = call-poly <vilib>:"CTRE_Phoenix_MotorController_Get_Enhanced.vi"("PhoenixMotorControlDevRef"=w242) -> ("Percent Output"=w203:dbl)  [unwired: 10 in, 4 out]
      "Percent Output 5" <- w203
      n89 = call-poly <vilib>:"CTRE_Phoenix_MotorController_Get_Enhanced.vi"("PhoenixMotorControlDevRef"=w242) -> ("Output Current"=w202:dbl)  [unwired: 12 in, 2 out]
      "Output Current 5" <- w202
      n90 = call-poly <vilib>:"CTRE_Phoenix_MotorController_Get_Enhanced.vi"("PhoenixMotorControlDevRef"=w225) -> ("Percent Output"=w204:dbl)  [unwired: 10 in, 4 out]
      "Percent Output 6" <- w204
      n91 = call-poly <vilib>:"CTRE_Phoenix_MotorController_Get_Enhanced.vi"("PhoenixMotorControlDevRef"=w225) -> ("Output Current"=w205:dbl)  [unwired: 12 in, 2 out]
      "Output Current 6" <- w205
      n92 = call-poly <vilib>:"CTRE_Phoenix_MotorController_Get_Enhanced.vi"("PhoenixMotorControlDevRef"=w242) -> ("Closed-loop Error"=w201:i32)  [unwired: 9 in, 5 out]
      "Closed-loop Error 5" <- w201
      n93 = call-poly <vilib>:"CTRE_Phoenix_MotorController_Get_Enhanced.vi"("PhoenixMotorControlDevRef"=w225) -> ("Closed-loop Error"=w200:i32)  [unwired: 9 in, 5 out]
      "Closed-loop Error 6" <- w200
      n94 = call-poly <vilib>:"CTRE_Phoenix_MotorController_Get_Enhanced.vi"("PhoenixMotorControlDevRef"=w242) -> ("Position (Raw Sensor Units)"=w199:i32, "Velocity (Raw Sensor Units per 100 ms)"=w191:i32, "error out"=w207:errorcluster)  [unwired: 11 in, 1 out]
      "Velocity (Raw Sensor Units per 100 ms) 7" <- w191
      "Position (Raw Sensor Units) 7" <- w199
      n95 = call-poly <vilib>:"CTRE_Phoenix_MotorController_Get_Enhanced.vi"("PhoenixMotorControlDevRef"=w225) -> ("Position (Raw Sensor Units)"=w187:i32, "Velocity (Raw Sensor Units per 100 ms)"=w190:i32, "error out"=w208:errorcluster)  [unwired: 11 in, 1 out]
      "Velocity (Raw Sensor Units per 100 ms) 8" <- w190
      "Position (Raw Sensor Units) 8" <- w187
      n96 = Subtract(x=w199, y=w187) -> (x-y=w198:i32)
      n97 = Merge Errors(w207, w208) -> (w206:errorcluster)
      n98 = call "Subvi_HowdyDrive_Teleop.vi"("error in (no error)"=w206, "Y axis value"=w189, "X axis value"=w188, "RobotDriveDevRef"=w197) -> ()  [unwired: 6 in, 2 out]
      n99 = Absolute Value(x=w198) -> (abs(x)=w196:i32)
      n100 = Bundle("Percent Output"=w203, "Output Current"=w202) -> (w194:T2)  [unwired: 1 in]
      n101 = Bundle("Closed-loop Error"=w201, "Closed-loop Error"=w200) -> (w195:T3)  [unwired: 1 in]
      n102 = Bundle(w189, "Velocity (Raw Sensor Units per 100 ms)"=w191, "Velocity (Raw Sensor Units per 100 ms)"=w190) -> (w192:T4)  [unwired: 1 in]
      n103 = Bundle("Percent Output"=w204, "Output Current"=w205) -> (w193:T2)  [unwired: 1 in]
    }
  }
  "encoder position" <- w26
  "closed loop error" <- w22
  "voltage vs current left" <- w25
  "Speed Closed Loop Plots" <- w24
  "voltage vs current right" <- w23
  n104 = Bundle(w13, "joystick Y Output"=w2) -> (→"X and Y":cluster{dbl, "joystick Y Output":dbl})  [unwired: 1 in]
  n105 = while {
    tunnel: w4 -> [w243]
    stop <- TRUE stop-if-true
    n106 = Divide(x=w243, y=2173 ("x")) -> (x/y=→"Position (inches) 6":dbl)
    "Position (Raw Sensor Units) 6" <- w243
  }
